vi "Analog_OutputMultipleChannels.vi"(8 "error in":errorcluster caption="entrée d'erreur") -> (0 "error out":errorcluster caption="sortie d'erreur")   [LabVIEW 2026]
uses:
  <userlib>/LV-Link3/PolySubVIs/DtCreateAoutChan.vi
panel:
  in  "Output voltage 0":dbl(slide) min=-10.0 max=10.0 step=0.1 scale=-10.0..10.0
  in  "Output voltage 1":dbl(slide) min=-10.0 max=10.0 step=0.1 scale=-10.0..10.0
  in  "stop":bool
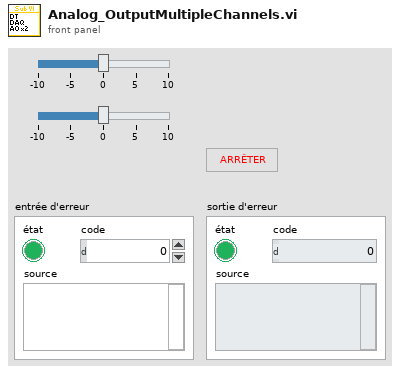
[diagram p1: front panel]
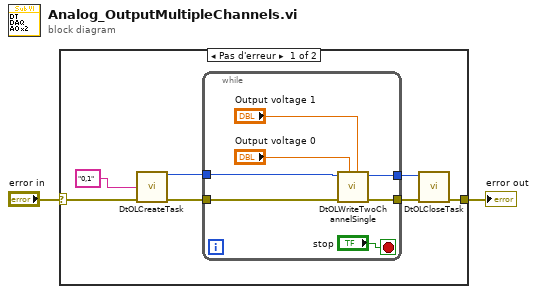
[diagram p0: block diagram]
diagram:
  n1 = case shown="Pas d'erreur" "error in" {
    selector: "error in" -> [w8 w17]
    tunnel: [w9 w17] -> w2
    frame No Error {
      n2 = call-poly <userlib>:"DtOLCreateTask.vi"("Channel"="0,1", "error in (no error)"=w8) -> ("Task out"=w6:i32, "error out"=w7:errorcluster)  [unwired: 11 in, 1 out]
      n3 = while {
        tunnel: w7 -> [w14]
        tunnel: w6 -> [w15]
        tunnel: [w13] -> w4
        tunnel: [w12] -> w3
        stop <- "stop" stop-if-true
        n4 = call <userlib>:"DtOLWriteTwoChannelSingle.vi"("Data for second channel"="Output voltage 1", "Data for first channel"="Output voltage 0", "error in (no error)"=w14, "Task in"=w15) -> ("error out"=w13:errorcluster, "Task out"=w12:i32)  [unwired: 6 in]
      }
      n5 = call <userlib>:"DtOLCloseTask.vi"("Error in"=w4, "Task in"=w3) -> ("Error Out"=w9:errorcluster)  [unwired: 9 in]
    }
    frame Error {
    }
  }
  "error out" <- w2
